vi "Pre-Build Action.vi"(6 "Top Level/Always Included VIs":path[](array[path]) caption="顶层/始终包括VI", 7 "Main Destination Path":path caption="主目标路径", 9 "Target Name":string caption="终端名称", 10 "Build Specification Name":string caption="程序生成规范名称", 11 "Project Path":path caption="项目路径") -> (0 "error out":errorcluster caption="错误输出")   [LabVIEW 2017]
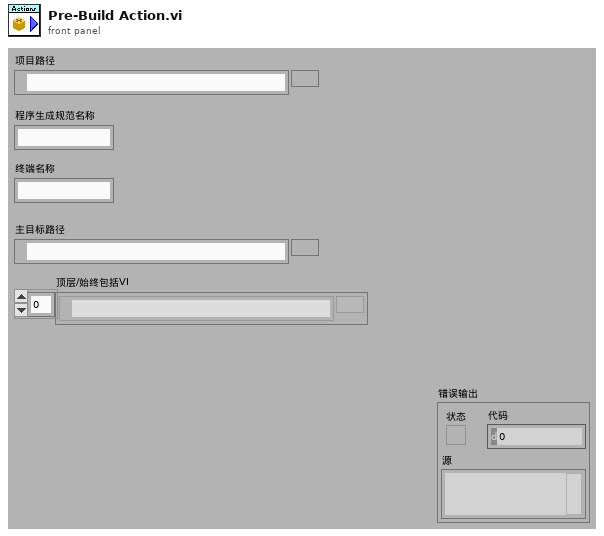
[diagram p1: front panel]
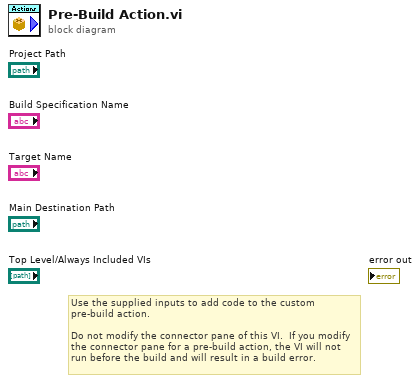
[diagram p0: block diagram]
diagram:
  # "Use the supplied inputs to add code to the custom pre-build action.\n\nDo not modify the connector pane of this VI.  If you modify the connector pane for a pre-build action, the VI will not run before the build and will result in a build error."
